vi "AddTestMethod_CreateNewWizard_Finalize.vi"(10 "Item":T1, 11 "Wizard":T1) -> ()   [LabVIEW 2013]
doc: "NI Confidential \n\n/**\n@brief This VI is called by the framework when an item of this type is first created.\n\n@author Joel Dixon\n\n@par Sample_Item_Init.vi\n This VI might typically set the popup menu for this item by calling mxLvSetPopupMenu.vi, set the icon for the item by calling mxLvSetIcon.vi, and set a name to be displayed in the tree by calling mxLvSetName.vi. \n\n@param \"Object\" [in] \nPassed by the framework as a reference to 'this' item in the tree. This parameter can be passed as the 'item' parameter for any of the mxLv** VIs, such as mxLvCreateItems.vi.\n*/"
uses:
  <resource>/Framework/Providers/API/ItemRef.ctl
  <resource>/Framework/Providers/API/mxLvUpdateUI.ctl
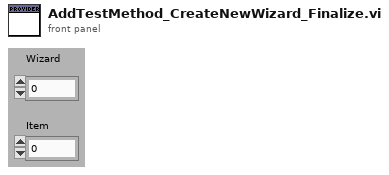
[diagram p1: front panel]
types:
  T1 = typedef "ItemRef.ctl" = u64
  T2 = typedef "mxLvUpdateUI.ctl" = cluster{"Action":u32, "Optional param 1":string, "Optional param 2":i32, "Optional param 3":string}
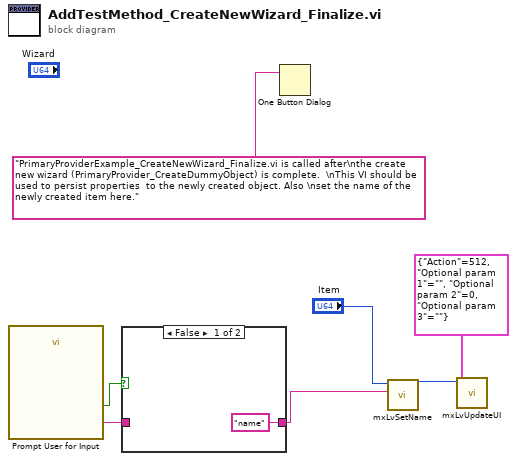
[diagram p0: block diagram]
diagram:
  n1 = call "Prompt User for Input"() -> ("Name"=w5:string, "OK"=w6:bool)  [unwired: 17 in, 1 out]
  n2 = case shown="False" w6 {
    tunnel: w5 -> [_ w9]
    tunnel: ["name" ("Name") w9] -> w3
    frame False {
    }
    frame True {
    }
  }
  n3 = One Button Dialog(message="PrimaryProviderExample_CreateNewWizard_Finalize.vi is called after\nthe create new wizard (PrimaryProvider_CreateDummyObject) is complete.  \nThis VI should be used to persist properties  to the newly created object. Also \nset the name of the newly created item here.") -> ()  [unwired: 1 in, 1 out]
  n4 = call <resource>:"mxLvSetName.vi"("Name"=w3, "Item"="Item") -> ("Item"=w2:T1)  [unwired: 8 in, 1 out]
  n5 = call <resource>:"mxLvUpdateUI.vi"("Update UI Settings"=T2 {"Action"=512, "Optional param 1"="", "Optional param 2"=0, "Optional param 3"=""}, "Item"=w2) -> ()  [unwired: 8 in, 2 out]
